vi "ReadHom2D.vi"(8 "error in (no error)":errorcluster caption="错误输入（无错误）") -> (0 "error out":errorcluster caption="错误输出", 1 "Robot":dbl[](array[numeric]), 2 "Camera":dbl[](array[numeric]), 3 "Snap":dbl[](array[numeric]))   [LabVIEW 2016]
uses:
  <vilib>/Utility/config.llb/Read Key (String).vi
  <vilib>/Utility/config.llb/NI_LVConfig.lvlib
  <vilib>/Utility/config.llb/Read Key (Double).vi
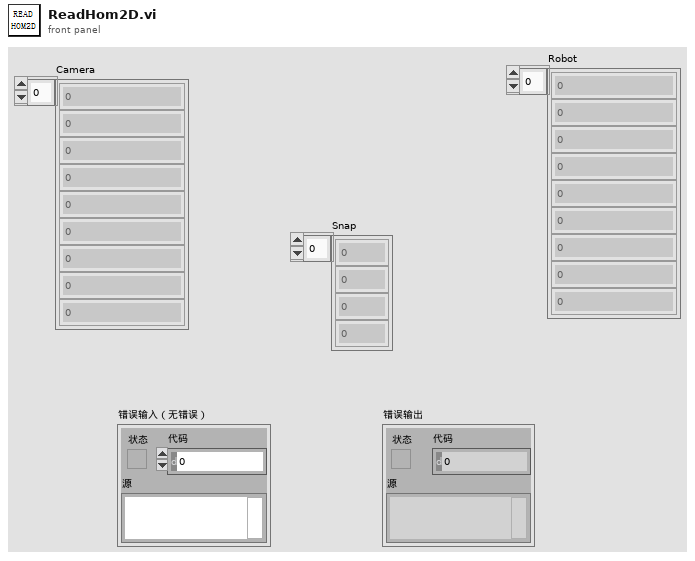
[diagram p1: front panel]
types:
  T1 = typedef "NI_LVConfig.lvlib/Config Data RefNum.ctl" = refnum<k1>
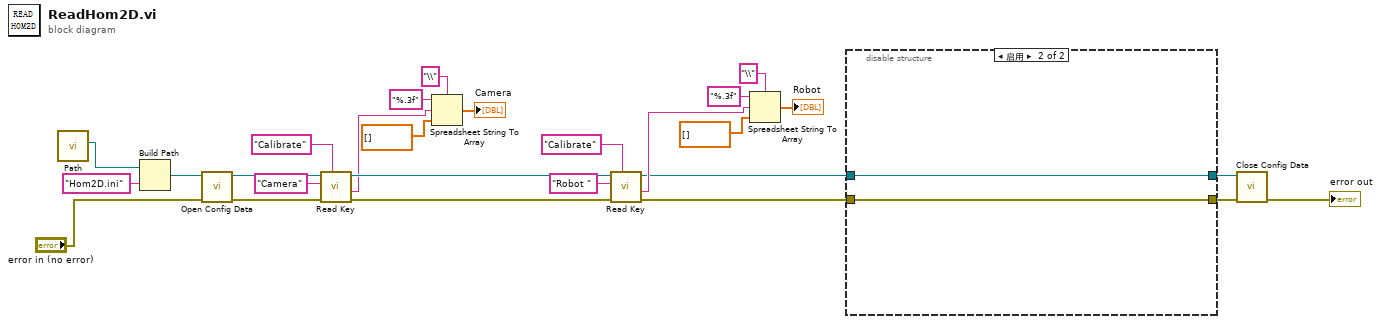
[diagram p0: block diagram]
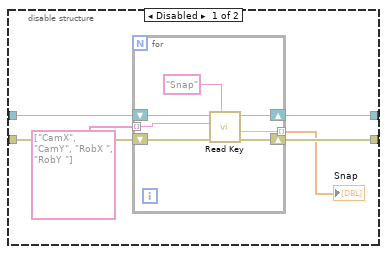
[diagram p2: hidden frame]
diagram:
  n1 = call "Path.vi"() -> ("Total"=w7:path)  [unwired: 11 in]
  n2 = Build Path(base path=w7, name or relative path="Hom2D.ini" ("名称或相对路径")) -> (appended path=w26:path)
  n3 = call <vilib>:"Open Config Data.vi"("error in (no error)"="error in (no error)", "configuration file path"=w26) -> ("error out"=w24:errorcluster, "refnum"=w25:T1)  [unwired: 7 in, 1 out]
  n4 = call-poly <vilib>:"Read Key.vi"("section"="Calibrate", "error in (no error)"=w24, "key"="Camera", "refnum"=w25) -> ("error out"=w18:errorcluster, "value"=w17:string, "refnum out"=w19:T1)  [unwired: 4 in, 1 out]
  n5 = Spreadsheet String To Array(delimiter (Tab)="\\" ("分隔符(Tab)"), format string="%.3f" ("格式字符串"), spreadsheet string=w17, array type (2D Dbl)=dbl[] []) -> (array=→"Camera":dbl[])
  n6 = call-poly <vilib>:"Read Key.vi"("section"="Calibrate", "error in (no error)"=w18, "key"="Robot ", "refnum"=w19) -> ("error out"=w5:errorcluster, "value"=w8:string, "refnum out"=w4:T1)  [unwired: 4 in, 1 out]
  n7 = Spreadsheet String To Array(delimiter (Tab)="\\" ("分隔符(Tab)"), format string="%.3f" ("格式字符串"), spreadsheet string=w8, array type (2D Dbl)=dbl[] []) -> (array=→"Robot":dbl[])
  n8 = disable-structure shown="启用" {
    disable-tunnel: [w33 w41] -> w6
    disable-tunnel: w5 -> [w32 w41]
    disable-tunnel: w4 -> [w31 w42]
    disable-tunnel: [w30 w42] -> w3
    frame Disabled {
      n9 = for {
        shift-right: [w39] -> w33
        shift-left: w32 -> [w38]
        shift-right: [w36] -> w30
        shift-left: w31 -> [w37]
        tunnel: string[] ["CamX", "CamY", "RobX ", "RobY "] -> [w35] mode=indexing
        tunnel: [w34] -> w28 mode=indexing
        n10 = call-poly <vilib>:"Read Key.vi"("section"="Snap", "error in (no error)"=w38, "key"=w35, "refnum"=w37) -> ("error out"=w39:errorcluster, "value"=w34:dbl, "refnum out"=w36:T1)  [unwired: 4 in, 1 out]
      }
      "Snap" <- w28
    }
    frame Enabled {
    }
  }
  n11 = call <vilib>:"Close Config Data.vi"("error in (no error)"=w6, "refnum"=w3) -> ("error out"=→"error out":errorcluster)  [unwired: 8 in, 1 out]
